vi "ResizeDemo.vi"() -> ()   [LabVIEW 2012]
uses:
  <vilib>/Utility/miscctls.llb/LVPointTypeDef.ctl
  <vilib>/Utility/cursorutil.llb/Set Cursor (Cursor ID).vi
  <vilib>/Utility/cursorutil.llb/Set Cursor (Icon Pict).vi
panel:
  out "波形图":dbl[](graph)
  in  "LBBorder":bool
  in  "RBBorder":bool
  in  "RTBorder":bool
  in  "LTBorder":bool
  in  "BottomBorder":bool
  in  "LeftBorder":bool
  in  "TopBorder":bool
  in  "Stop":bool
  in  "RightBorder":bool
  in  "Title":bool
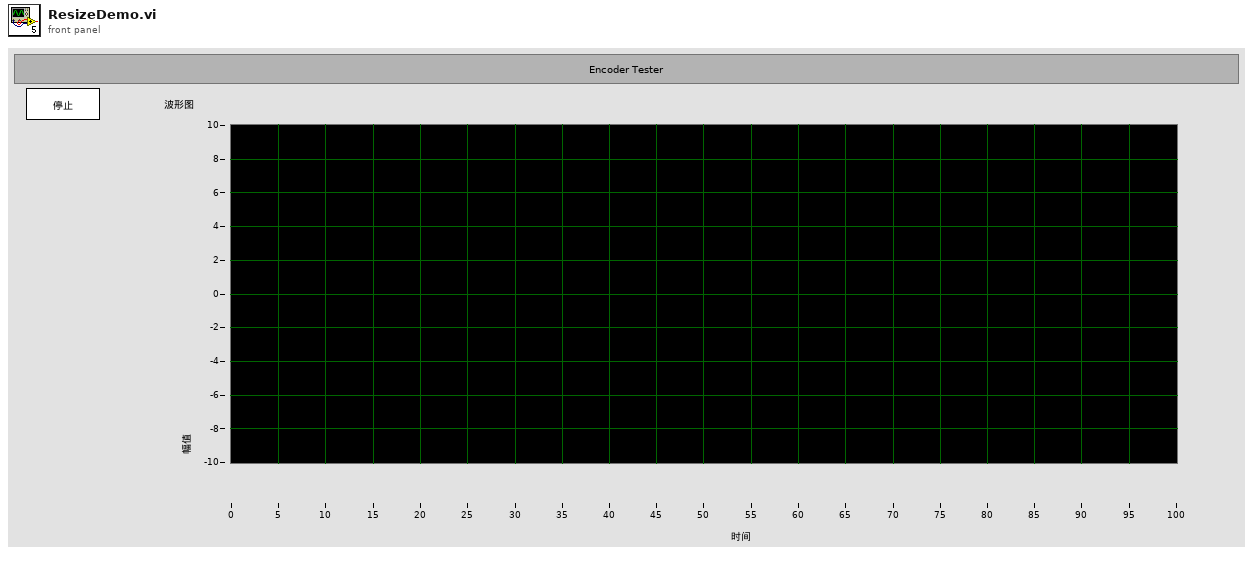
[diagram p1: front panel]
types:
  T1 = typedef "LVPointTypeDef.ctl" = cluster{"Horizontal":i16, "Vertical":i16}
  T2 = cluster{"LeftBorder":refnum<vi>, "TopBorder":refnum<vi>, "RightBorder":refnum<vi>, "BottomBorder":refnum<vi>, "本VI":refnum<vi>, "Title":refnum<vi>, "LTBorder":refnum<vi>, "RTBorder":refnum<vi>, "RBBorder":refnum<vi>, "LBBorder":refnum<vi>}
  T3 = enum32{"Invalid", "Standard", "Closed", "Hidden", "Minimized", "Maximized"}
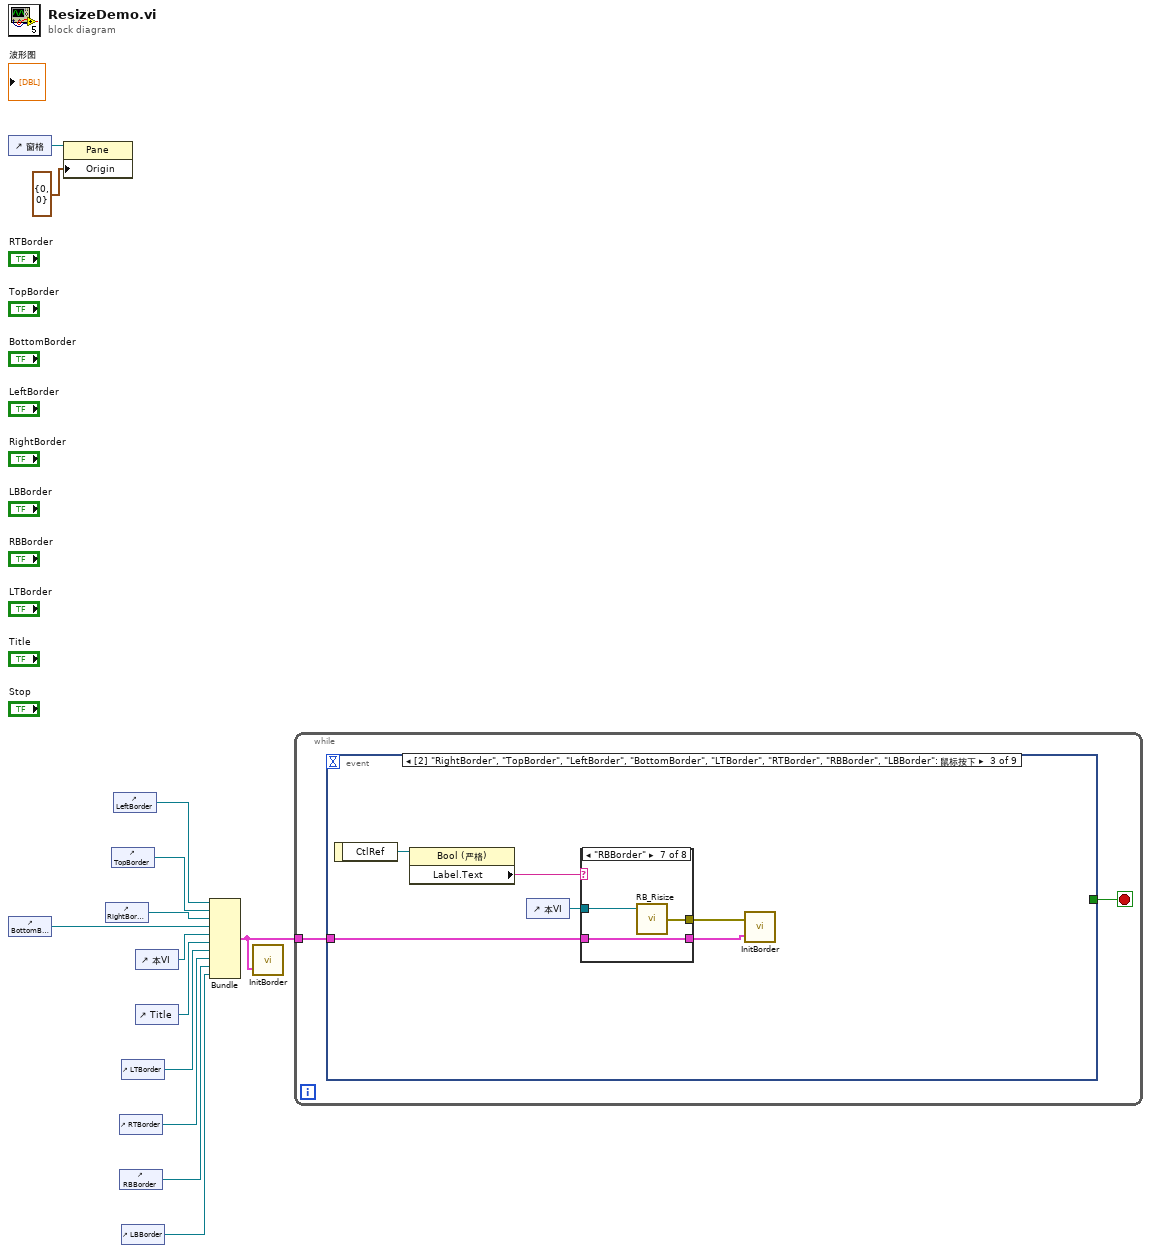
[diagram p0: block diagram]
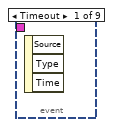
[diagram p2: hidden frame]
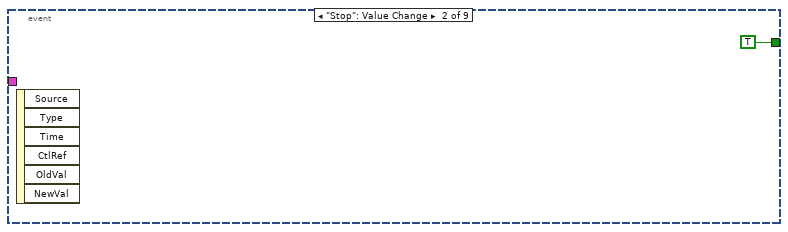
[diagram p3: hidden frame]
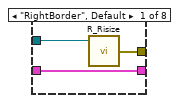
[diagram p4: hidden frame]
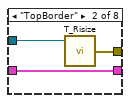
[diagram p5: hidden frame]
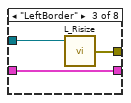
[diagram p6: hidden frame]
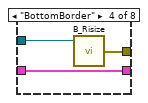
[diagram p7: hidden frame]
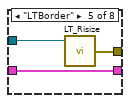
[diagram p8: hidden frame]
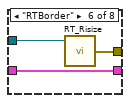
[diagram p9: hidden frame]
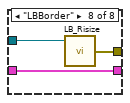
[diagram p10: hidden frame]
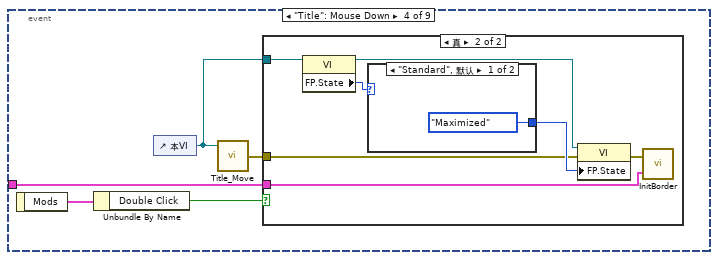
[diagram p11: hidden frame]
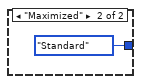
[diagram p13: hidden frame]
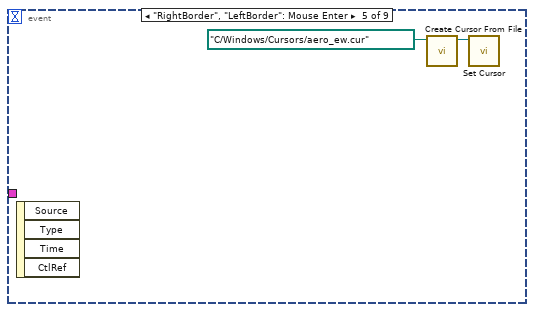
[diagram p14: hidden frame]
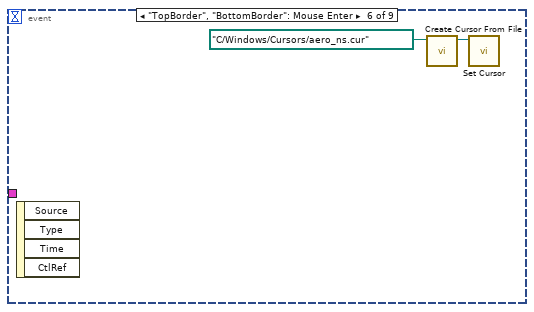
[diagram p15: hidden frame]
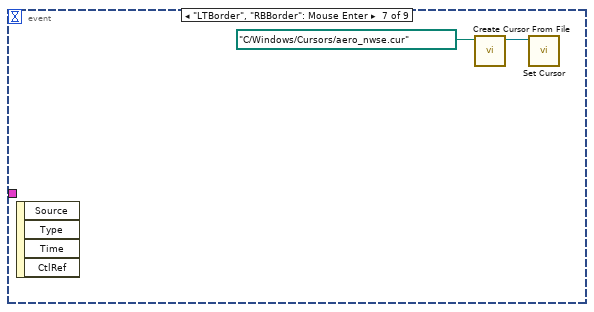
[diagram p16: hidden frame]
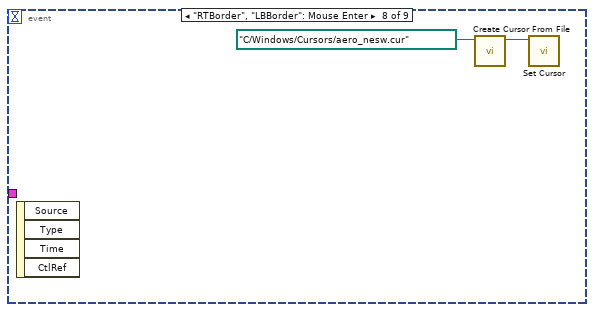
[diagram p17: hidden frame]
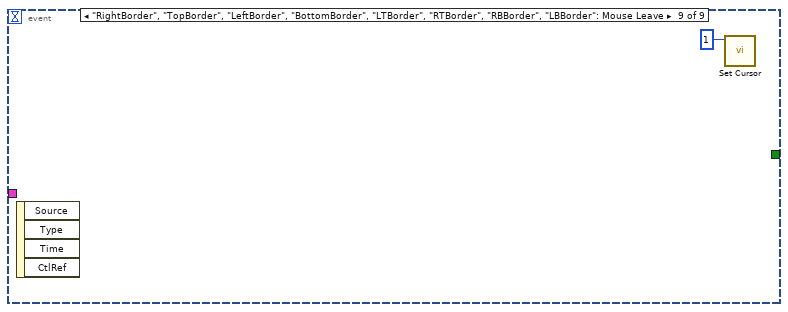
[diagram p18: hidden frame]
diagram:
  n1 = control-ref of="窗格"() -> (w12:refnum<vi>)
  n2 = control-ref of="BottomBorder"() -> (w6:refnum<vi>)
  n3 = property on="属性节点" class="Pane"(reference=w12, "Origin"=T1 {"Horizontal"=0, "Vertical"=0} ("原点")) -> ()  [unwired: 1 in, 2 out]
  n4 = control-ref of="RightBorder"() -> (w5:refnum<vi>)
  n5 = control-ref of="TopBorder"() -> (w4:refnum<vi>)
  n6 = control-ref of="LeftBorder"() -> (w3:refnum<vi>)
  n7 = control-ref of="RTBorder"() -> (w9:refnum<vi>)
  n8 = control-ref of="RBBorder"() -> (w10:refnum<vi>)
  n9 = control-ref of="LTBorder"() -> (w8:refnum<vi>)
  n10 = control-ref of="LBBorder"() -> (w2:refnum<vi>)
  n11 = control-ref of="本VI"() -> (w7:refnum<vi>)
  n12 = control-ref of="Title"() -> (w11:refnum<vi>)
  n13 = Bundle("LeftBorder"=w3, "TopBorder"=w4, "RightBorder"=w5, "BottomBorder"=w6, "本VI"=w7, "Title"=w11, "LTBorder"=w8, "RTBorder"=w9, "RBBorder"=w10, "LBBorder"=w2) -> (w1:T2)  [unwired: 1 in]
  n14 = call "InitBorder.vi"("引用簇"=w1) -> ()  [unwired: 1 in, 1 out]
  n15 = while {
    tunnel: w1 -> [w14]
    stop <- w15 stop-if-true
    n16 = event shown="[2] \"RightBorder\", \"TopBorder\", \"LeftBorder\", \"BottomBorder\", \"LTBorder\", \"RTBorder\", \"RBBorder\", \"LBBorder\": 鼠标按下" {
      selector: _ -> [_ _ _ _ _ _ _ _ _]
      dyn-events: _ -> [_ _ _ _ _ _ _ _ _]
      timeout: _ -> [_ _ _ _ _ _ _ _ _]
      tunnel: [_ TRUE _ _ _ _ _ _ _] -> w15
      tunnel: w14 -> [_ _ w20 w48 _ _ _ _ _]
      event Timeout {
        n17 = event-data() -> ()  [unwired: 1 in, 3 out]
      }
      event "Stop": Value Change {
        n18 = event-data() -> ()  [unwired: 1 in, 6 out]
      }
      event "RightBorder", "TopBorder", "LeftBorder", "BottomBorder", "LTBorder", "RTBorder", "RBBorder", "LBBorder": Mouse Down {
        n19 = event-data() -> ("CtlRef"=w22:refnum<vi>)  [unwired: 1 in]
        n20 = property class="Bool (严格)"(reference=w22) -> ("Label.Text"=w21:string)  [unwired: 1 in, 2 out]
        n21 = control-ref of="本VI"() -> (w17:refnum<vi>)
        n22 = case shown="\"RBBorder\"" w21 {
          tunnel: w20 -> [w25 w28 w29 w32 w35 w39 w42 w44]
          tunnel: [w25 w28 w29 w32 w35 w39 w42 w44] -> w19
          tunnel: [w24 w27 w31 w34 w36 w40 w43 w46] -> w18
          tunnel: w17 -> [w23 w26 w30 w33 w37 w38 w41 w45]
          frame "RightBorder", Default {
            n23 = call "R_Risize.vi"("本VI"=w23) -> ("error out"=w24:errorcluster)  [unwired: 2 in]
          }
          frame "TopBorder" {
            n24 = call "T_Risize.vi"("本VI"=w26) -> ("error out"=w27:errorcluster)  [unwired: 2 in]
          }
          frame "LeftBorder" {
            n25 = call "L_Risize.vi"("本VI"=w30) -> ("error out"=w31:errorcluster)  [unwired: 2 in]
          }
          frame "BottomBorder" {
            n26 = call "B_Risize.vi"("本VI"=w33) -> ("error out"=w34:errorcluster)  [unwired: 2 in]
          }
          frame "LTBorder" {
            n27 = call "LT_Risize.vi"("本VI"=w37) -> ("error out"=w36:errorcluster)  [unwired: 2 in]
          }
          frame "RTBorder" {
            n28 = call "RT_Risize.vi"("本VI"=w38) -> ("error out"=w40:errorcluster)  [unwired: 2 in]
          }
          frame "RBBorder" {
            n29 = call "RB_Risize.vi"("本VI"=w41) -> ("error out"=w43:errorcluster)  [unwired: 2 in]
          }
          frame "LBBorder" {
            n30 = call "LB_Risize.vi"("本VI"=w45) -> ("error out"=w46:errorcluster)  [unwired: 2 in]
          }
        }
        n31 = call "InitBorder.vi"("引用簇"=w19, "error in (no error)"=w18) -> ()  [unwired: 1 out]
      }
      event "Title": Mouse Down {
        n32 = event-data() -> ("Mods"=w51:cluster{"Double Click":bool, "Menu Key":bool})  [unwired: 1 in]
        n33 = Unbundle By Name(w51) -> ("Double Click"=w50:bool)
        n34 = control-ref of="本VI"() -> (w47:refnum<vi>)
        n35 = call "Title_Move.vi"("本VI"=w47) -> ("error out"=w49:errorcluster)  [unwired: 2 in]
        n36 = case shown="真" w50 {
          tunnel: w49 -> [_ w57]
          tunnel: w48 -> [_ w55]
          tunnel: w47 -> [_ w53]
          frame False {
          }
          frame True {
            n37 = property class="VI"(reference=w53) -> (reference out=w52:refnum<vi>, "FP.State"=w56:T3)  [unwired: 1 in, 1 out]
            n38 = case shown="\"Standard\", 默认" w56 {
              tunnel: [T3."Maximized" ("前面板窗口:状态") T3."Standard" ("前面板窗口:状态")] -> w58
              frame "Standard", Default {
              }
              frame "Maximized" {
              }
            }
            n39 = property class="VI"(reference=w52, error in=w57, "FP.State"=w58) -> (error out=w54:errorcluster)  [unwired: 1 out]
            n40 = call "InitBorder.vi"("引用簇"=w55, "error in (no error)"=w54) -> ()  [unwired: 1 out]
          }
        }
      }
      event "RightBorder", "LeftBorder": Mouse Enter {
        n41 = event-data() -> ()  [unwired: 1 in, 4 out]
        n42 = call <vilib>:"Create Cursor From File.vi"("cursor file"=path "C:/Windows/Cursors/aero_ew.cur") -> ("cursor ID"=w62:refnum<k1>)  [unwired: 9 in, 1 out]
        n43 = call-poly <vilib>:"Set Cursor.vi"("cursor ID"=w62) -> ()  [unwired: 9 in, 2 out]
      }
      event "TopBorder", "BottomBorder": Mouse Enter {
        n44 = event-data() -> ()  [unwired: 1 in, 4 out]
        n45 = call <vilib>:"Create Cursor From File.vi"("cursor file"=path "C:/Windows/Cursors/aero_ns.cur") -> ("cursor ID"=w64:refnum<k1>)  [unwired: 9 in, 1 out]
        n46 = call-poly <vilib>:"Set Cursor.vi"("cursor ID"=w64) -> ()  [unwired: 9 in, 2 out]
      }
      event "LTBorder", "RBBorder": Mouse Enter {
        n47 = event-data() -> ()  [unwired: 1 in, 4 out]
        n48 = call <vilib>:"Create Cursor From File.vi"("cursor file"=path "C:/Windows/Cursors/aero_nwse.cur") -> ("cursor ID"=w66:refnum<k1>)  [unwired: 9 in, 1 out]
        n49 = call-poly <vilib>:"Set Cursor.vi"("cursor ID"=w66) -> ()  [unwired: 9 in, 2 out]
      }
      event "RTBorder", "LBBorder": Mouse Enter {
        n50 = event-data() -> ()  [unwired: 1 in, 4 out]
        n51 = call <vilib>:"Create Cursor From File.vi"("cursor file"=path "C:/Windows/Cursors/aero_nesw.cur") -> ("cursor ID"=w68:refnum<k1>)  [unwired: 9 in, 1 out]
        n52 = call-poly <vilib>:"Set Cursor.vi"("cursor ID"=w68) -> ()  [unwired: 9 in, 2 out]
      }
      event "RightBorder", "TopBorder", "LeftBorder", "BottomBorder", "LTBorder", "RTBorder", "RBBorder", "LBBorder": Mouse Leave {
        n53 = event-data() -> ()  [unwired: 1 in, 4 out]
        n54 = call-poly <vilib>:"Set Cursor.vi"("icon"=u16 1) -> ()  [unwired: 9 in, 2 out]
      }
    }
  }
